vi "TC_to_DSC.vi"(6 "AVS names":T2={"AVS Name 0"="3K", "AVS Name 1"="Still", "AVS Name 2"="50 mK", "AVS Name 3"="MC", "AVS Name 4"="MC", "AVS Name 5"="", "AVS Name 6"="", "AVS Name 7"="", "AVS Name 8"="", "AVS Name 9"=""}, 7 "AVS type":T1(ring) caption="Bridge Type", 8 "Array":refnum<vi>[](array[refnum]), 9 "I":dbl[](array[numeric]), 10 "T":dbl[](array[numeric]), 11 "R":dbl[](array[numeric])) -> ()   [LabVIEW 2016]
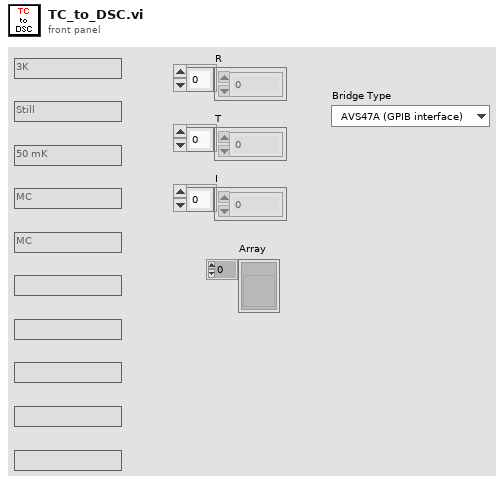
[diagram p1: front panel]
types:
  T1 = enum16{"AVS47A (GPIB interface)", "AVS47B (RS232 interface)", "AVS48", "AVS Emulation", "Impedance Bridge", "Disabled"}
  T2 = cluster{"AVS Name 0":string, "AVS Name 1":string, "AVS Name 2":string, "AVS Name 3":string, "AVS Name 4":string, "AVS Name 5":string, "AVS Name 6":string, "AVS Name 7":string, "AVS Name 8":string, "AVS Name 9":string}
  T3 = cluster{"[0]":string, "[1]":string, "[2]":string, "[3]":string, "[4]":string, "[5]":string, "[6]":string, "[7]":string, "[8]":string, "[9]":string}
  T4 = enum16{"CF", "CF_Z_Bridge", "MNK", "MNK_Z_Bridge"}
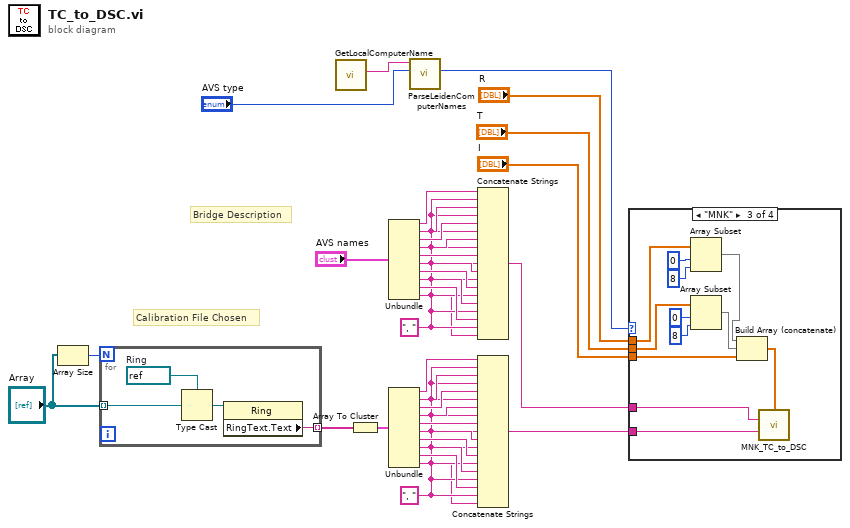
[diagram p0: block diagram]
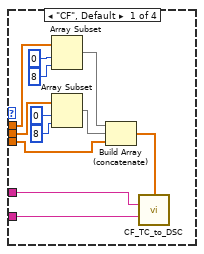
[diagram p2: hidden frame]
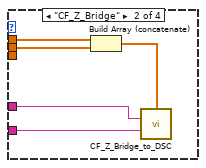
[diagram p3: hidden frame]
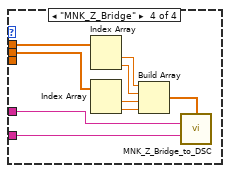
[diagram p4: hidden frame]
diagram:
  w11 = ", " ("string")
  w25 = ", " ("string")
  # "Bridge Description"
  # "Calibration File Chosen"
  n1 = Array Size(array="Array") -> (size(s)=w22:i32)
  n2 = for {
    N: w22 -> [_]
    tunnel: "Array" -> [w39] mode=indexing
    tunnel: [w36] -> w21 mode=indexing
    w38 = refnum<vi> refnum  # Ring
    n3 = Type Cast(type=w38, x=w39) -> (*(type *) &x=w37:refnum<vi>)
    n4 = property class="Ring"(reference=w37) -> ("RingText.Text"=w36:string)  [unwired: 1 in, 2 out]
  }
  n5 = call "GetLocalComputerName.vi"() -> ("Name"=w1:string)  [unwired: 10 in, 1 out]
  n6 = Array To Cluster(array=w21) -> (cluster=w9:T3)
  n7 = Unbundle("AVS names") -> ("AVS Name 0"=w34:string, "AVS Name 1"=w33:string, "AVS Name 2"=w32:string, "AVS Name 3"=w31:string, "AVS Name 4"=w30:string, "AVS Name 5"=w29:string, "AVS Name 6"=w28:string, "AVS Name 7"=w27:string, "AVS Name 8"=w26:string, "AVS Name 9"=w24:string)
  n8 = Unbundle(w9) -> ("[0]"=w20:string, "[1]"=w19:string, "[2]"=w18:string, "[3]"=w17:string, "[4]"=w16:string, "[5]"=w15:string, "[6]"=w14:string, "[7]"=w13:string, "[8]"=w12:string, "[9]"=w10:string)
  n9 = call "ParseLeidenComputerNames.vi"("AVS type"="AVS type", "computer name"=w1) -> ("AVS Type"=w5:T4)  [unwired: 7 in, 2 out]
  n10 = Concatenate Strings(w34, w25, w33, w25, w32, w25, w31, w25, w30, w25, w29, w25, w28, w25, w27, w25, w26, w25, w24) -> (w23:string)
  n11 = Concatenate Strings(w20, w11, w19, w11, w18, w11, w17, w11, w16, w11, w15, w11, w14, w11, w13, w11, w12, w11, w10) -> (w7:string)
  n12 = case shown="\"MNK\"" w5 {
    tunnel: "R" -> [w40 w56 w60 w76]
    tunnel: "T" -> [w43 w55 w59 w77]
    tunnel: "I" -> [w44 _ w68 _]
    tunnel: w23 -> [w51 w54 w66 w70]
    tunnel: w7 -> [w50 w53 w67 w69]
    frame "CF", Default {
      n13 = Array Subset(array=w40, index=0, length=8) -> (w42:dbl[])
      n14 = Array Subset(array=w43, index=0, length=8) -> (w41:dbl[])
      n15 = Build Array (concatenate)(w42, w41, w44) -> (w49:dbl[])
      n16 = call "CF_TC_to_DSC.vi"("dbl"=w49, "String In"=w51, "String In 2"=w50) -> ()  [unwired: 12 in, 1 out]
    }
    frame "CF_Z_Bridge" {
      n17 = Build Array (concatenate)(w56, w55) -> (w52:dbl[])
      n18 = call "CF_Z_Bridge_to_DSC.vi"("dbl"=w52, "String In"=w54, "String In 2"=w53) -> ()  [unwired: 12 in, 1 out]
    }
    frame "MNK" {
      n19 = Array Subset(array=w60, index=0, length=8) -> (w57:dbl[])
      n20 = Array Subset(array=w59, index=0, length=8) -> (w58:dbl[])
      n21 = Build Array (concatenate)(w57, w58, w68) -> (w65:dbl[])
      n22 = call "MNK_TC_to_DSC.vi"("dbl"=w65, "String In"=w66, "String In 2"=w67) -> ()  [unwired: 12 in, 1 out]
    }
    frame "MNK_Z_Bridge" {
      n23 = Index Array(array=w76) -> (element #1=w75:dbl, element #2=w74:dbl)  [unwired: 2 in]
      n24 = Index Array(array=w77) -> (element #1=w73:dbl, element #2=w72:dbl)  [unwired: 2 in]
      n25 = Build Array(w75, w74, w73, w72) -> (w71:dbl[])
      n26 = call "MNK_Z_Bridge_to_DSC.vi"("dbl"=w71, "String In"=w70, "String In 2"=w69) -> ()  [unwired: 13 in]
    }
  }
